vi "CodigoLabView 1_1.vi"() -> ()   [LabVIEW 2025]
uses:
  <vilib>/Instr/_visa.llb/VISA Configure Serial Port (Instr).vi
panel:
  in  "Relé N°4":bool
  in  "Relé N°3":bool
  in  "Relé N°2":bool
  in  "Relé N°1":bool
  out "Serial Settings:Number of Bytes at Serial Port":u32
  out "error out 2":errorcluster
  out "Enviando":string
  out "error out":errorcluster
  out "Meter":dbl(knob) scale=0.0..5.0 scale format="%#_6f"
  out "Numeric":dbl
  out "String":string
  in  "VISA resource name":refnum<visa-resource-name>
  in  "stop":bool
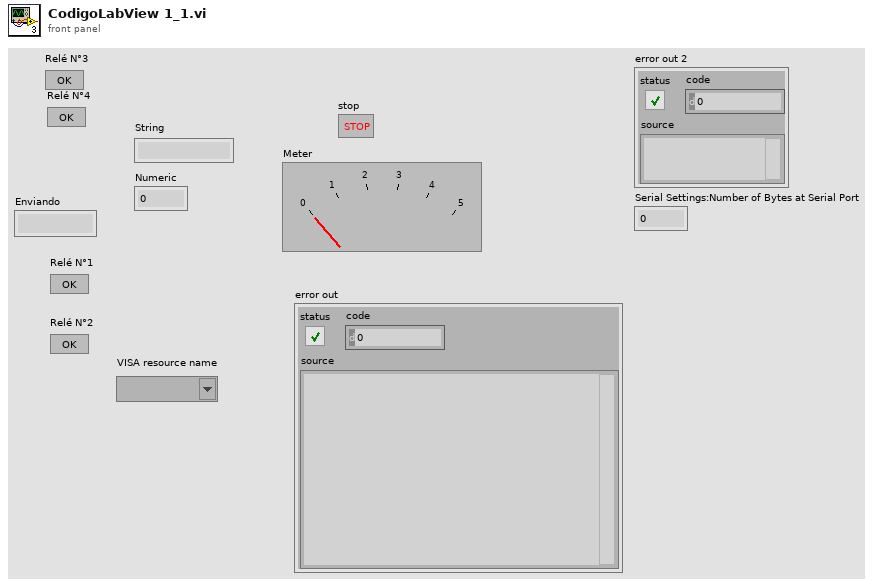
[diagram p1: front panel]
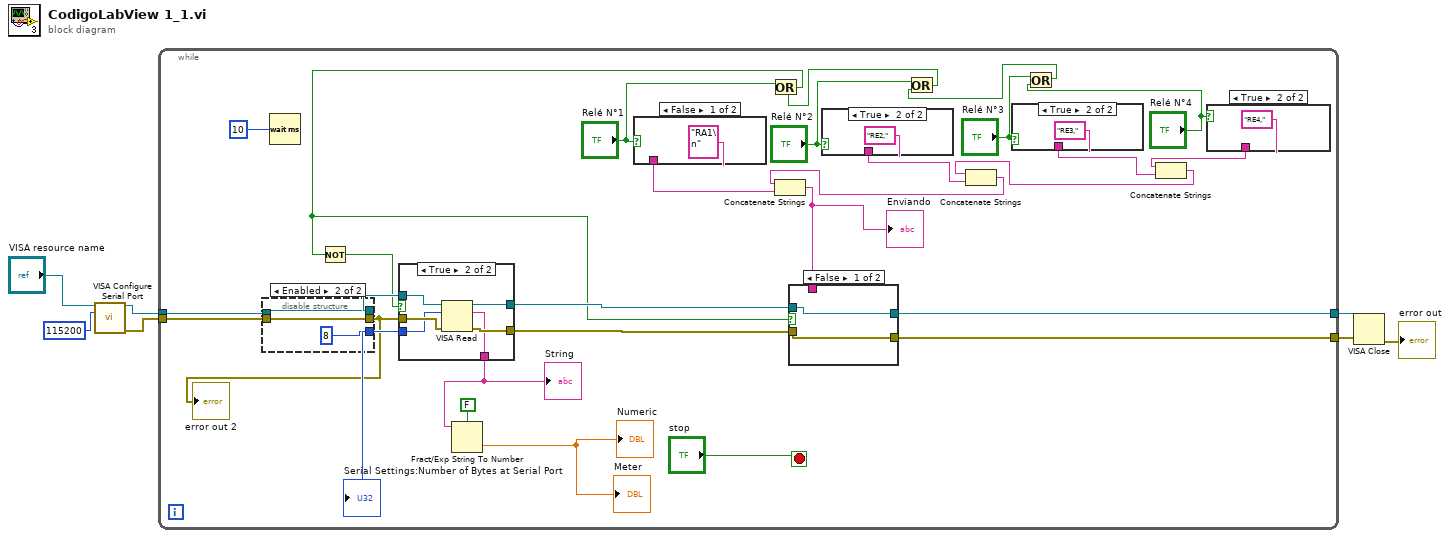
[diagram p0: block diagram]
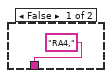
[diagram p2: hidden frame]
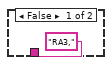
[diagram p3: hidden frame]
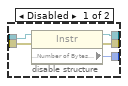
[diagram p4: hidden frame]
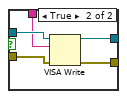
[diagram p6: hidden frame]
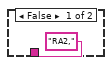
[diagram p7: hidden frame]
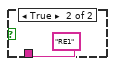
[diagram p8: hidden frame]
diagram:
  n1 = call-poly "VISA Configure Serial Port"("VISA resource name"="VISA resource name", "baud rate (9600)"=u32 115200) -> ("VISA resource name out"=w7:refnum<visa-resource-name>, "error out"=w1:errorcluster)  [unwired: 12 in]
  n2 = while {
    tunnel: w7 -> [w35]
    tunnel: [w30] -> w6
    tunnel: w1 -> [w34]
    tunnel: [w29] -> w5
    stop <- "stop" stop-if-true
    n3 = disable-structure shown="Enabled" {
      disable-tunnel: w35 -> [w45 w48]
      disable-tunnel: w34 -> [w44 w47]
      disable-tunnel: [w43 w48] -> w26
      disable-tunnel: [w42 u32 8 ("Bytes at Port")] -> w25
      disable-tunnel: [w41 w47] -> w23
      frame Disabled {
        n4 = property class="Instr"(reference=w45, error in=w44) -> (reference out=w43:refnum<visa-resource-name>, error out=w41:errorcluster, "Serial Settings:Number of Bytes at Serial Port"=w42:u32)
      }
      frame Enabled {
      }
    }
    "error out 2" <- w23
    "Serial Settings:Number of Bytes at Serial Port" <- w25
    n5 = Wait (ms)(milliseconds to wait=u32 10) -> ()  [unwired: 1 out]
    n6 = case shown="False" "Relé N°1" {
      tunnel: ["RA1\n" "RE1"] -> w31
      frame False {
      }
      frame True {
      }
    }
    n7 = case shown="True" "Relé N°2" {
      tunnel: ["RA2," "RE2,"] -> w10
      frame False {
      }
      frame True {
      }
    }
    n8 = case shown="True" "Relé N°3" {
      tunnel: ["RA3," "RE3,"] -> w12
      frame False {
      }
      frame True {
      }
    }
    n9 = Or(x="Relé N°3", y="Relé N°4") -> (x .or. y?=w17:bool)
    n10 = Or(x="Relé N°2", y=w17) -> (x .or. y?=w14:bool)
    n11 = Or(x="Relé N°1", y=w14) -> (x .or. y?=w21:bool)
    n12 = Not(x=w21) -> (.not. x?=w22:bool)
    n13 = case shown="True" w22 {
      tunnel: [w50 w56] -> w28
      tunnel: [w49 w55] -> w27
      tunnel: w23 -> [w49 w54]
      tunnel: w26 -> [w50 w53]
      tunnel: w25 -> [_ w52]
      tunnel: [_ w51] -> w24
      frame False {
      }
      frame True {
        n14 = VISA Read(VISA resource name=w53, byte count=w52, error in (no error)=w54) -> (VISA resource name out=w56:refnum<visa-resource-name>, read buffer=w51:string, error out=w55:errorcluster)  [unwired: 1 out]
      }
    }
    "String" <- w24
    n15 = Fract/Exp String To Number(use system decimal point (T)=FALSE, string=w24) -> (number=→"Numeric" →"Meter":dbl)  [unwired: 2 in, 1 out]
    n16 = case shown="True" "Relé N°4" {
      tunnel: ["RA4," "RE4,"] -> w13
      frame False {
      }
      frame True {
      }
    }
    n17 = Concatenate Strings(w13, w12) -> (w11:string)
    n18 = Concatenate Strings(w11, w10) -> (w9:string)
    n19 = Concatenate Strings(w9, w31) -> (w8:string)
    "Enviando" <- w8
    n20 = case shown="False" w21 {
      tunnel: [w58 w63] -> w30
      tunnel: [w57 w62] -> w29
      tunnel: w28 -> [w58 w61]
      tunnel: w27 -> [w57 w60]
      tunnel: w8 -> [_ w59]
      frame False {
      }
      frame True {
        n21 = VISA Write(VISA resource name=w61, write buffer=w59, error in (no error)=w60) -> (VISA resource name out=w63:refnum<visa-resource-name>, error out=w62:errorcluster)  [unwired: 1 out]
      }
    }
  }
  n22 = VISA Close(VISA resource name=w6, error in (no error)=w5) -> (error out=→"error out":errorcluster)
